vi "Get register for reading - single.vi"(11 "Reg in":string) -> (3 "Reg out":string)   [LabVIEW 2020, in "Toggle 8.lvclass"]
uses:
  Toggle 8.lvclass
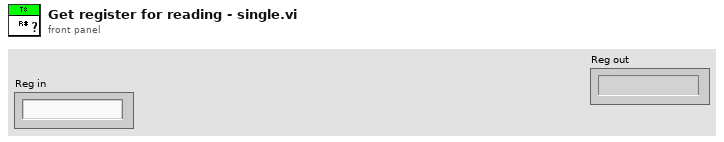
[diagram p1: front panel]
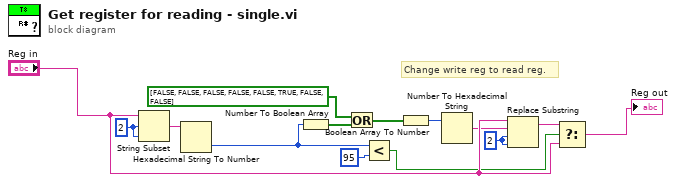
[diagram p0: block diagram]
diagram:
  w6 = 2 ("offset (0)")
  w5 = 2 ("length (rest)")
  # "Change write reg to read reg."
  n1 = String Subset(string="Reg in", offset (0)=w5, length (rest)=w5) -> (substring=w8:string)
  n2 = Hexadecimal String To Number(string=w8) -> (number=w4:u32)  [unwired: 2 in, 1 out]
  n3 = Number To Boolean Array(number=w4) -> (Boolean array=w11:bool[])
  n4 = Or(x=bool[] [FALSE, FALSE, FALSE, FALSE, FALSE, TRUE, FALSE, FALSE] ("Boolean array"), y=w11) -> (x .or. y?=w10:bool[])
  n5 = Less?(x=w4, y=u32 95) -> (x < y?=w2:bool)
  n6 = Boolean Array To Number(Boolean array=w10) -> (number=w9:u32)
  n7 = Number To Hexadecimal String(2:w9) -> (0:w7:string)  [unwired: 1 in]
  n8 = Replace Substring(2:w6, 3:w6, 4:w7, 5:"Reg in") -> (1:w1:string)  [unwired: 1 out]
  n9 = Select(t=w1, s=w2, f="Reg in") -> (s? t:f=→"Reg out":string)
